vi "modem1.vi"() -> ()   [LabVIEW 2010]
uses:
  <vilib>/Instr/_visa.llb/VISA Configure Serial Port (Instr).vi
panel:
  out "DCD":bool
  out "RI":bool
  out "DSR":bool
  out "CTS":bool=TRUE
  out "DTR state":bool
  out "RTS state":bool
  in  "RTS":bool
  in  "DTR":bool
  in  "Write to DTR and RTS?":bool=TRUE
  in  "VISA resource name":refnum<visa-resource-name>="COM1"
  in  "line index":i32
  in  "OK Button 2":bool
  in  "multi-line string":string="at+cfun=1\nat+wipcfg=1\nat+wipbr=1,6\nat+wipbr=2,6,11,\"internet\"\nat+wipbr=2,6,0,\"\"\nat+wipbr=2,6,1,\"\"\nat+wipbr=4,6,0\nat+wipcreate=4,1,\"ftp.newmail.ru\",21,\"test2011\",\"123456\"\nat+wipfile=4,1,2,\"./test1.txt\"\n456544687846545678745uuuu\nat+wipbr=5,6\nat+wipbr=0,6\nat+wipcfg=0"
  in  "OK Button":bool
  out "String":string
  in  "stop":bool
  out "error out":errorcluster
  out "read buffer":string
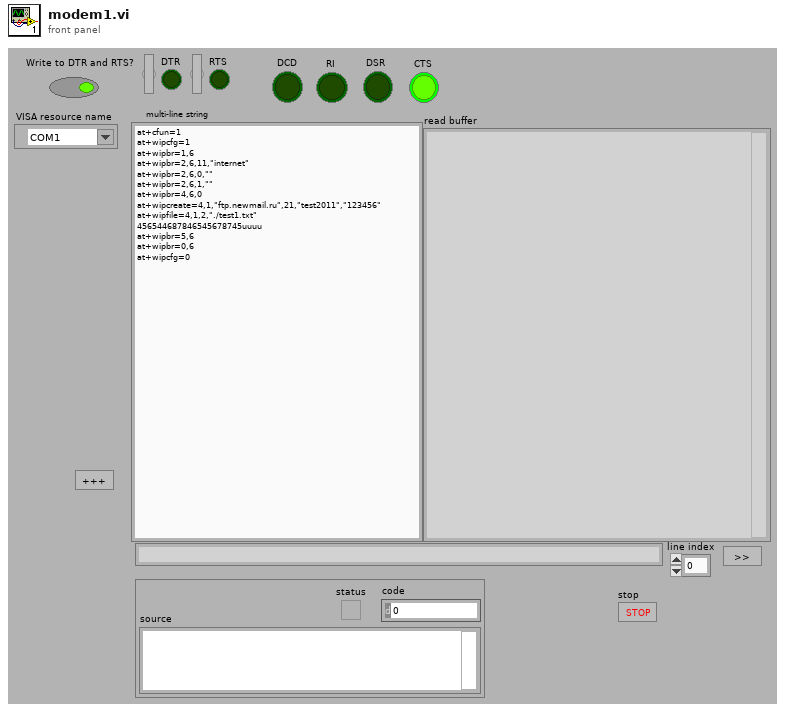
[diagram p1: front panel]
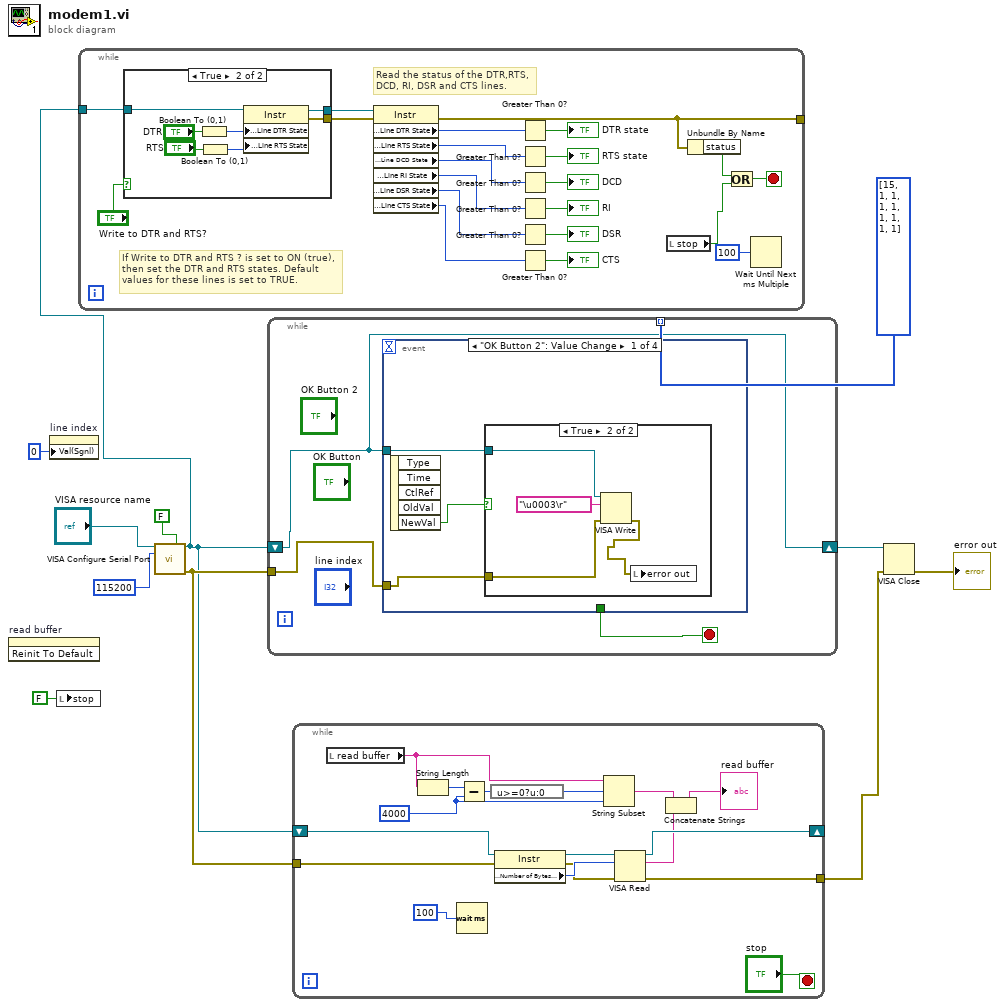
[diagram p0: block diagram]
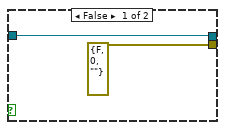
[diagram p2: hidden frame]
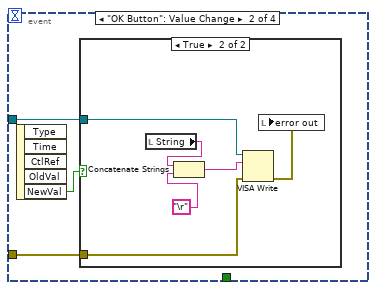
[diagram p4: hidden frame]
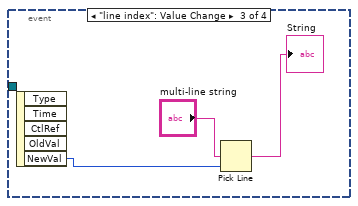
[diagram p6: hidden frame]
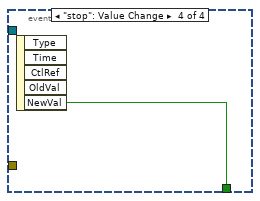
[diagram p7: hidden frame]
diagram:
  n1 = invoke on="read buffer" class="Str" method="Reinit To Default"() -> ()  [unwired: 3 in, 3 out]
  n2 = property on="line index" class="DigNum (strict)"("Val(Sgnl)"=0 ("Value (Signaling)")) -> ()  [unwired: 2 in, 2 out]
  n3 = local write "stop"(FALSE ("stop")) -> ()
  n4 = call-poly "VISA Configure Serial Port"("VISA resource name"="VISA resource name", "Enable Termination\nChar (T)"=FALSE ("Enable Termination\nChar (T)"), "baud rate (9600)"=u32 115200) -> ("VISA resource name out"=w1:refnum<visa-resource-name>, "error out"=w6:errorcluster)  [unwired: 11 in]
  n5 = while {
    tunnel: w1 -> [w31]
    tunnel: [w30] -> _
    stop <- w32 stop-if-true
    # "Read the status of the DTR,RTS,\nDCD, RI, DSR and CTS lines."
    # "If Write to DTR and RTS ? is set to ON (true), then set the DTR and RTS states. Default values for these lines is set to TRUE."
    n6 = case shown="True" "Write to DTR and RTS?" {
      tunnel: w31 -> [w34 w40]
      tunnel: [w34 w36] -> w29
      tunnel: [errorcluster {"status"=FALSE, "code"=0, "source"=""} ("error in (no error)") w35] -> w28
      frame False {
      }
      frame True {
        n7 = Boolean To (0,1)(Boolean="DTR") -> (0, 1=w37:i16)
        n8 = Boolean To (0,1)(Boolean="RTS") -> (0, 1=w39:i16)
        n9 = property class="Instr"(reference=w40, "Serial Settings:Modem Line Settings:Line DTR State"=w37, "Serial Settings:Modem Line Settings:Line RTS State"=w39) -> (reference out=w36:refnum<visa-resource-name>, error out=w35:errorcluster)  [unwired: 1 in]
      }
    }
    n10 = property class="Instr"(reference=w29, error in=w28) -> (error out=w30:errorcluster, "Serial Settings:Modem Line Settings:Line DTR State"=w24:i16, "Serial Settings:Modem Line Settings:Line RTS State"=w20:i16, "Serial Settings:Modem Line Settings:Line DCD State"=w21:i16, "Serial Settings:Modem Line Settings:Line RI State"=w27:i16, "Serial Settings:Modem Line Settings:Line DSR State"=w26:i16, "Serial Settings:Modem Line Settings:Line CTS State"=w25:i16)  [unwired: 1 out]
    n11 = Greater Than 0?(x=w24) -> (x > 0?=→"DTR state":bool)
    n12 = Greater Than 0?(x=w20) -> (x > 0?=→"RTS state":bool)
    n13 = Greater Than 0?(x=w21) -> (x > 0?=→"DCD":bool)
    n14 = Greater Than 0?(x=w27) -> (x > 0?=→"RI":bool)
    n15 = Greater Than 0?(x=w26) -> (x > 0?=→"DSR":bool)
    n16 = Greater Than 0?(x=w25) -> (x > 0?=→"CTS":bool)
    n17 = local read "stop"() -> (w12:bool)
    n18 = Unbundle By Name(w30) -> ("status"=w13:bool)
    n19 = Or(x=w13, y=w12) -> (x .or. y?=w32:bool)
    n20 = Wait Until Next ms Multiple(millisecond multiple=u32 100) -> ()  [unwired: 1 out]
  }
  n21 = while {
    shift-right: [w42] -> w7
    shift-left: w1 -> [w42]
    tunnel: u32[] [15, 1, 1, 1, 1, 1, 1, 1, 1] -> [_] mode=indexing
    tunnel: w6 -> [w43]
    stop <- w44 stop-if-true
    n22 = event shown="[0] \"OK Button 2\": Value Change" {
      selector: _ -> [_ _ _ _]
      dyn-events: _ -> [_ _ _ _]
      timeout: _ -> [_ _ _ _]
      tunnel: w42 -> [w46 w53 _ _]
      tunnel: [_ _ _ w64] -> w44
      tunnel: w43 -> [w45 w52 _ _]
      event "OK Button 2": Value Change {
        n23 = event-data() -> ("NewVal"=w47:bool)  [unwired: 1 in, 4 out]
        n24 = case shown="True" w47 {
          tunnel: w46 -> [_ w50]
          tunnel: w45 -> [_ w49]
          frame False {
          }
          frame True {
            n25 = VISA Write(VISA resource name=w50, write buffer="\u0003\r", error in (no error)=w49) -> (error out=w48:errorcluster)  [unwired: 2 out]
            n26 = local write "error out"(w48) -> ()
          }
        }
      }
      event "OK Button": Value Change {
        n27 = event-data() -> ("NewVal"=w54:bool)  [unwired: 1 in, 4 out]
        n28 = case shown="True" w54 {
          tunnel: w53 -> [_ w58]
          tunnel: w52 -> [_ w57]
          frame False {
          }
          frame True {
            n29 = local read "String"() -> (w55:string)
            n30 = Concatenate Strings(w55, "\r") -> (w59:string)
            n31 = VISA Write(VISA resource name=w58, write buffer=w59, error in (no error)=w57) -> (error out=w56:errorcluster)  [unwired: 2 out]
            n32 = local write "error out"(w56) -> ()
          }
        }
      }
      event "line index": Value Change {
        n33 = event-data() -> ("NewVal"=w62:i32)  [unwired: 1 in, 4 out]
        n34 = Pick Line(multi-line string="multi-line string", line index=w62) -> (output string=→"String":string)  [unwired: 1 in]
      }
      event "stop": Value Change {
        n35 = event-data() -> ("NewVal"=w64:bool)  [unwired: 1 in, 4 out]
      }
    }
  }
  n36 = while {
    shift-right: [w78] -> _
    shift-left: w1 -> [w77]
    tunnel: w6 -> [w76]
    tunnel: [w75] -> w3
    stop <- "stop" stop-if-true
    w71 = 4000 ("length (rest)")
    n37 = local read "read buffer"() -> (w73:string)
    n38 = String Length(string=w73) -> (length=w72:i32)
    n39 = Wait (ms)(milliseconds to wait=u32 100) -> ()  [unwired: 1 out]
    n40 = Subtract(x=w72, y=w71) -> (x-y=w65:i32)
    n41 = expression code="u>=0?u:0"(w65) -> (w66:i32)
    n42 = property class="Instr"(reference=w77, error in=w76) -> (reference out=w79:refnum<visa-resource-name>, error out=w80:errorcluster, "Serial Settings:Number of Bytes at Serial Port"=w81:u32)
    n43 = String Subset(string=w73, offset (0)=w66, length (rest)=w71) -> (substring=w69:string)
    n44 = VISA Read(VISA resource name=w79, byte count=w81, error in (no error)=w80) -> (VISA resource name out=w78:refnum<visa-resource-name>, read buffer=w68:string, error out=w75:errorcluster)  [unwired: 1 out]
    n45 = Concatenate Strings(w69, w68) -> (→"read buffer":string)
  }
  n46 = VISA Close(VISA resource name=w7, error in (no error)=w3) -> (error out=→"error out":errorcluster)
